vi "20220114_Dialog.vi"() -> ()   [LabVIEW 2019]
panel:
  in  "確定":bool
  in  "Name":string
  # "請輸入你的英文名字"
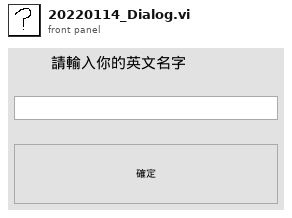
[diagram p1: front panel]
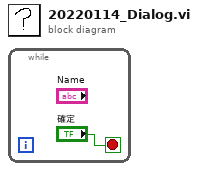
[diagram p0: block diagram]
diagram:
  n1 = while {
    stop <- "確定" stop-if-true
  }
